vi "GetName.vi"(8 "error in (no error)":errorcluster caption="错误输入（无错误）", 11 "TCPClientClass 输入":refnum<class "TCPClientClass.lvclass">) -> (0 "error out":errorcluster caption="错误输出", 2 "结果字符串":string, 3 "TCPClientClass 输出":refnum<class "TCPClientClass.lvclass">)   [LabVIEW 2019, in "TCPClientClass.lvclass"]
uses:
  TCPClientClass.lvclass
  TCPClientClass.lvclass/TCPClientClass.ctl
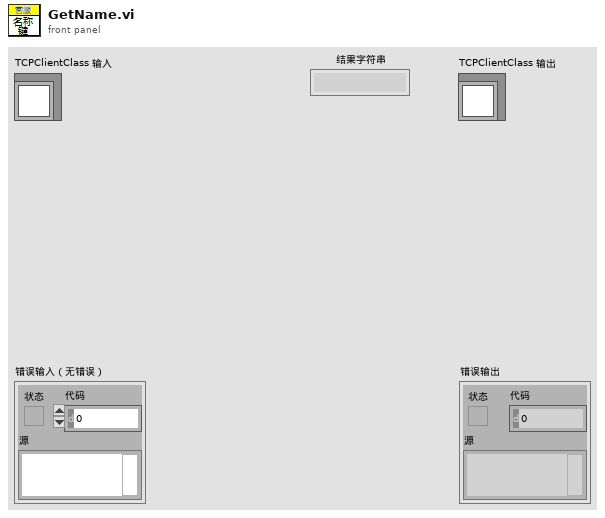
[diagram p1: front panel]
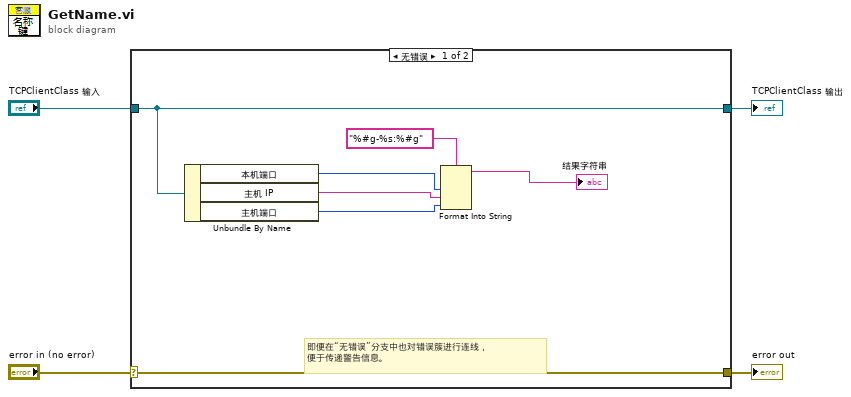
[diagram p0: block diagram]
diagram:
  n1 = case shown="无错误" "error in (no error)" {
    selector: "error in (no error)" -> [w11 w13]
    tunnel: [w11 w13] -> w3
    tunnel: [w10 w12] -> w1
    tunnel: "TCPClientClass 输入" -> [w10 w12]
    frame No Error {
      # "即便在“无错误”分支中也对错误簇进行连线，\n便于传递警告信息。"
      n2 = Unbundle By Name(w10) -> ("本机端口"=w8:u16, "主机 IP"=w7:string, "主机端口"=w6:u16)
      n3 = Format Into String(format string="%#g-%s:%#g" ("格式字符串"), w8, w7, w6) -> (resulting string=→"结果字符串":string)  [unwired: 2 in, 1 out]
    }
    frame Error {
    }
  }
  "error out" <- w3
  "TCPClientClass 输出" <- w1
